vi "FTW-App-StringVersionToString.vi"(8 "Build":string, 9 "Fix":string, 10 "Minor":string, 11 "Major":string) -> (1 "Version String (minus Build)":string, 2 "Version String":string)   [LabVIEW 2015]
panel:
  # "Inputs"
  # "Outputs"
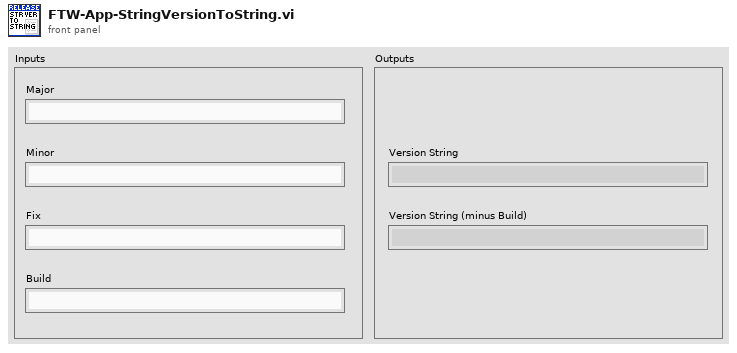
[diagram p1: front panel]
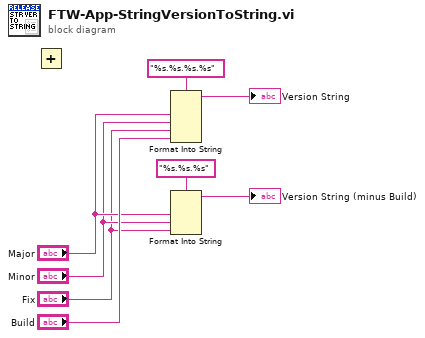
[diagram p0: block diagram]
diagram:
  n1 = Add() -> ()  [unwired: 2 in, 1 out]
  n2 = Format Into String(format string="%s.%s.%s.%s", "Major", "Minor", "Fix", "Build") -> (resulting string=→"Version String":string)  [unwired: 2 in, 1 out]
  n3 = Format Into String(format string="%s.%s.%s", "Major", "Minor", "Fix") -> (resulting string=→"Version String (minus Build)":string)  [unwired: 2 in, 1 out]
